vi "SSL Geometry Data.vi"(5 "Version":string(combo)="Auto", 7 "Optional":bool, 8 "error in":errorcluster, 9 "Array":u8[](array[numeric]) format="%02x") -> (0 "error out":errorcluster, 2 "Geometry Camera Calibration":T1, 3 "Field Size":T2)   [LabVIEW 2017]
uses:
  SSL Geometry Camera Calibration.ctl
  Varint Decoder uint32.vi
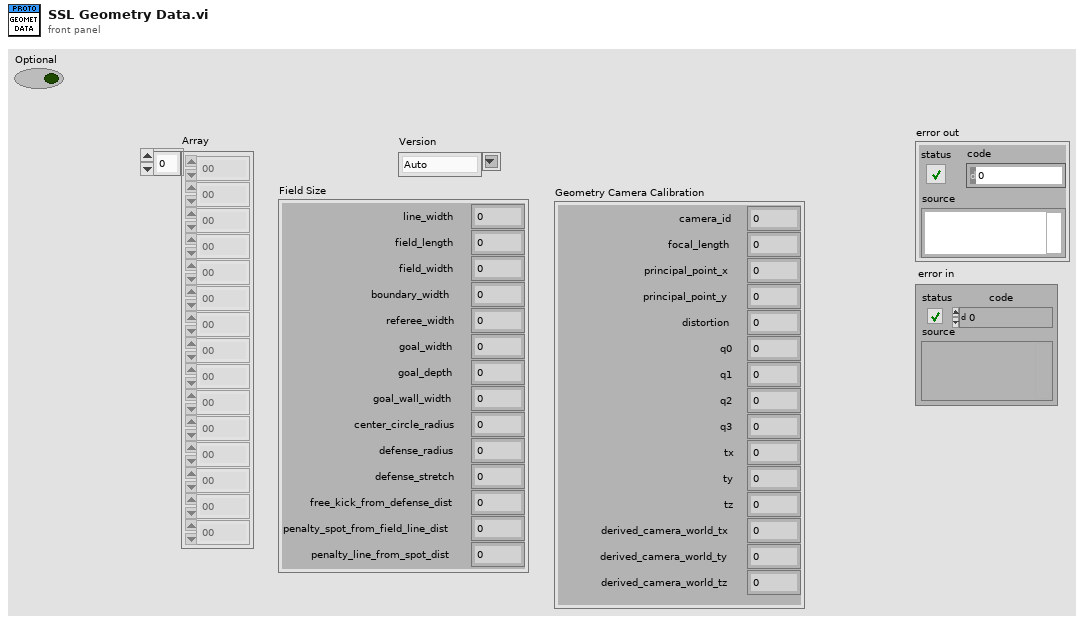
[diagram p1: front panel]
types:
  T1 = typedef "SSL Geometry Camera Calibration.ctl" = cluster{"camera_id":u32, "focal_length":sgl, "principal_point_x":sgl, "principal_point_y":sgl, "distortion":sgl, "q0":sgl, "q1":sgl, "q2":sgl, "q3":sgl, "tx":sgl, "ty":sgl, "tz":sgl, "derived_camera_world_tx":sgl, "derived_camera_world_ty":sgl, "derived_camera_world_tz":sgl}
  T2 = cluster{"line_width":u32, "field_length":u32, "field_width":u32, "boundary_width":u32, "referee_width":u32, "goal_width":u32, "goal_depth":u32, "goal_wall_width":u32, "center_circle_radius":u32, "defense_radius":u32, "defense_stretch":u32, "free_kick_from_defense_dist":u32, "penalty_spot_from_field_line_dist":u32, "penalty_line_from_spot_dist":u32}
  T3 = cluster{"[0]":sgl, "[1]":sgl, "[2]":sgl, "[3]":sgl, "[4]":sgl, "[5]":sgl, "[6]":sgl, "[7]":sgl, "[8]":sgl, "[9]":sgl, "[10]":sgl, "[11]":sgl, "[12]":sgl, "[13]":sgl, "[14]":sgl}
  T4 = cluster{"[0]":u32, "[1]":u32, "[2]":u32, "[3]":u32, "[4]":u32, "[5]":u32, "[6]":u32, "[7]":u32, "[8]":u32, "[9]":u32, "[10]":u32, "[11]":u32, "[12]":u32, "[13]":u32}
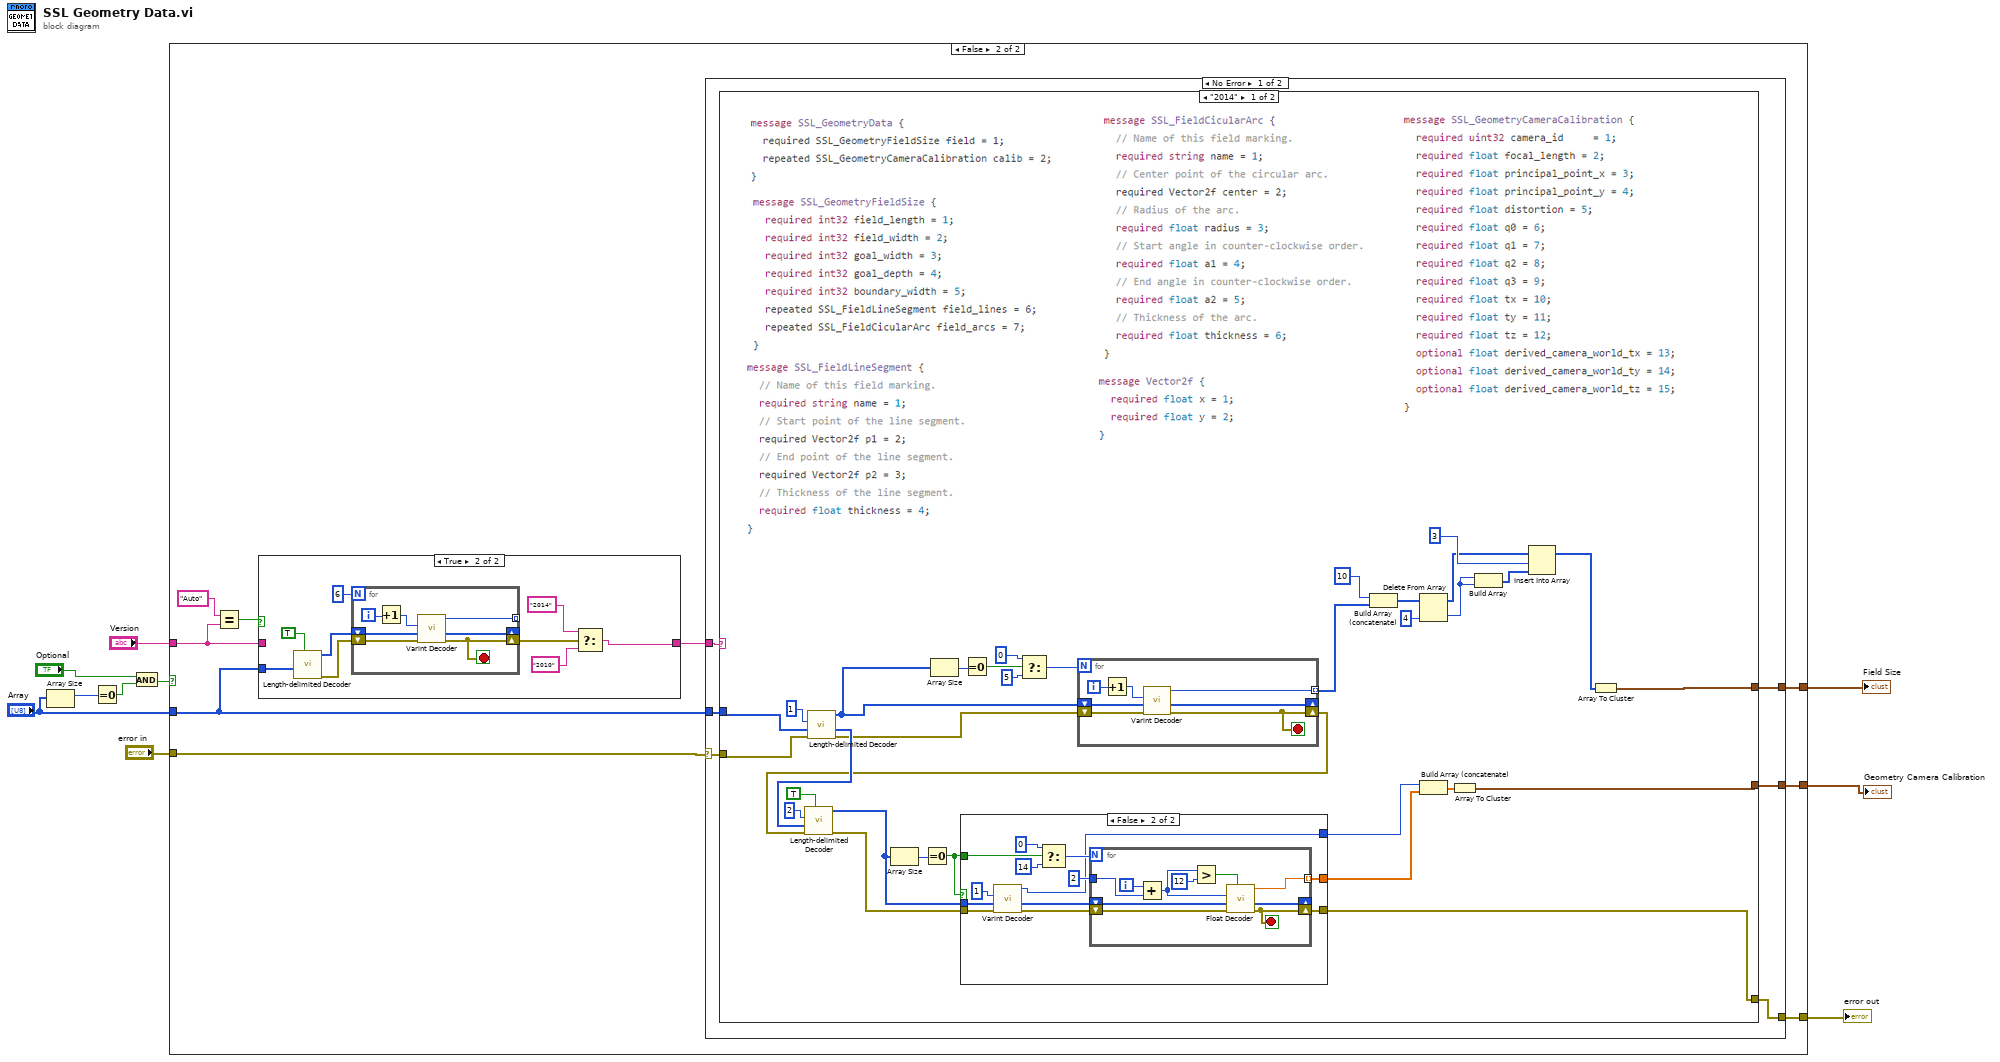
[diagram p0: block diagram]
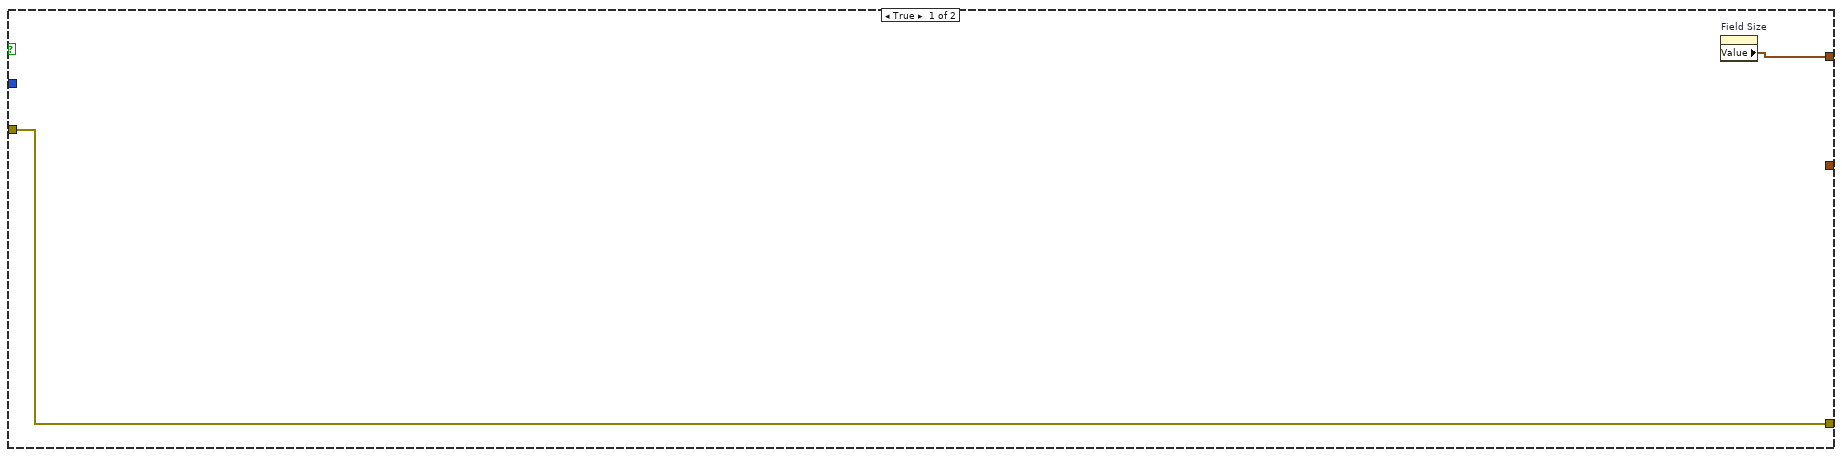
[diagram p2: hidden frame]
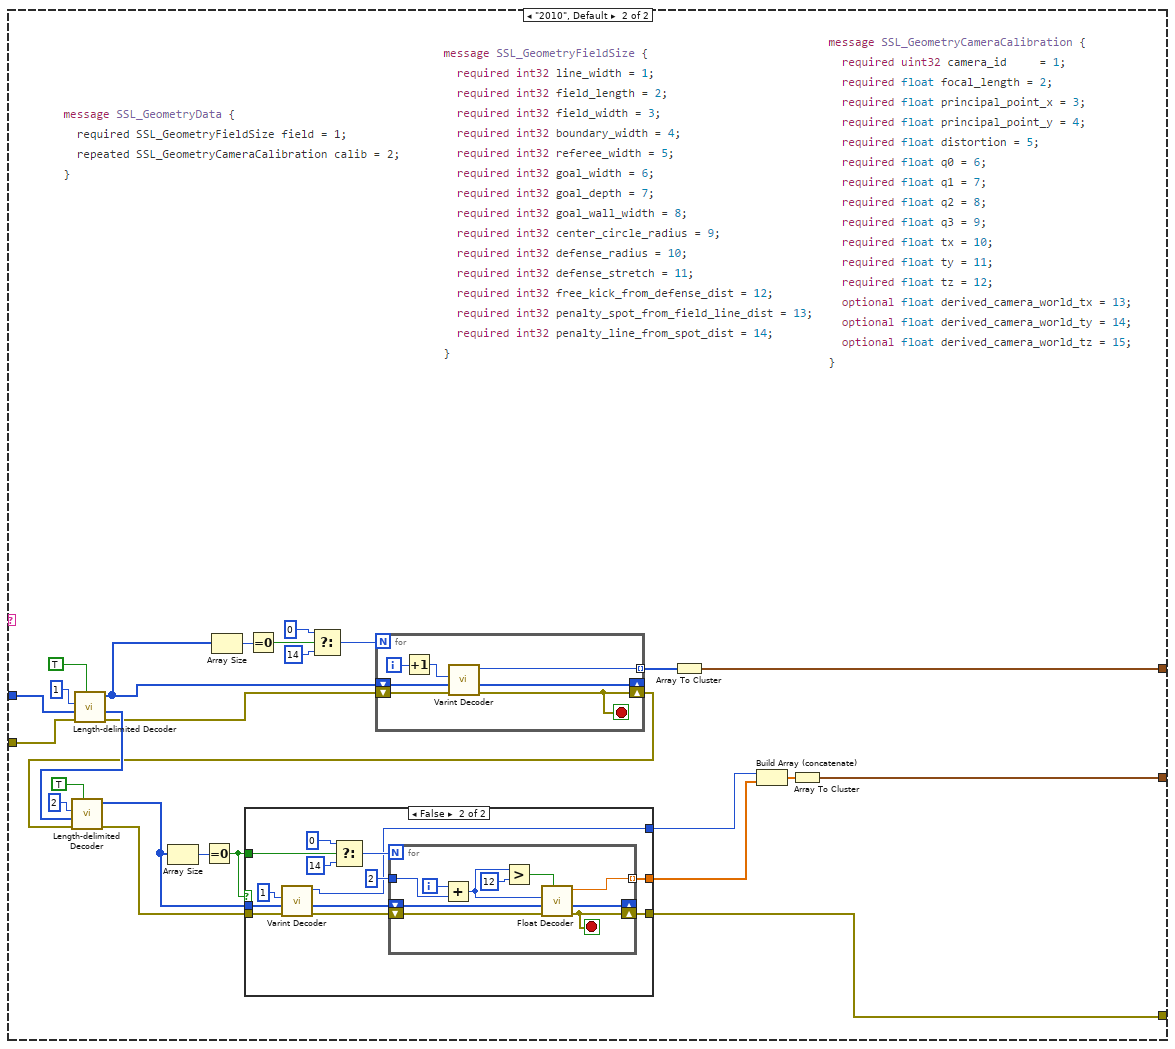
[diagram p5: hidden frame]
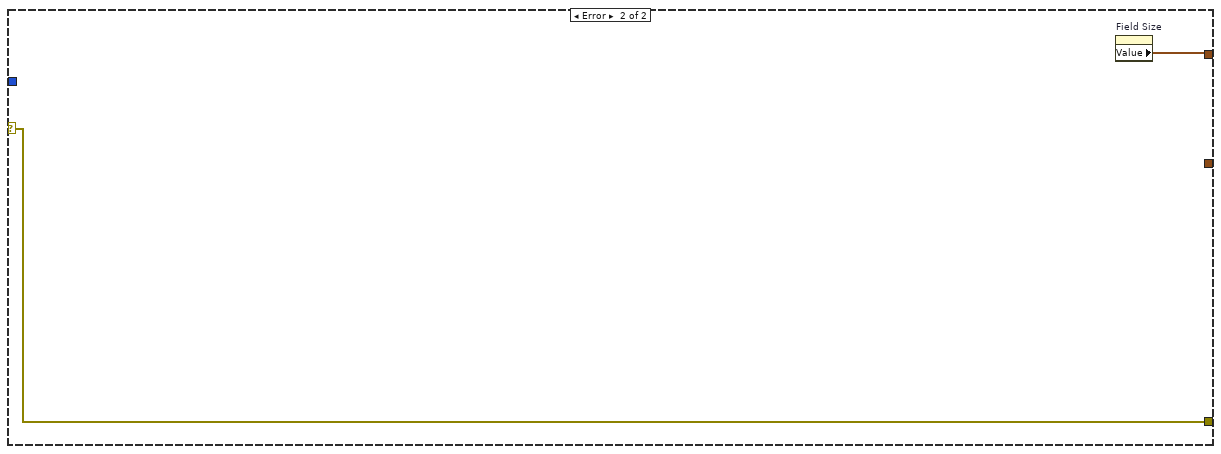
[diagram p7: hidden frame]
diagram:
  n1 = Array Size(array="Array") -> (size(s)=w4:i32)
  n2 = Equal To 0?(x=w4) -> (x = 0?=w5:bool)
  n3 = And(x="Optional", y=w5) -> (x .and. y?=w6:bool)
  n4 = case shown="False" w6 {
    tunnel: "error in" -> [w12 w21]
    tunnel: [w12 w20] -> w9
    tunnel: "Array" -> [_ w13]
    tunnel: "Version" -> [_ w15]
    tunnel: [w11 w19] -> w2
    tunnel: [_ w18] -> w1
    frame True {
      n5 = property on="Field Size" class="Clust (strict)"() -> ("Value"=w11:T2)  [unwired: 2 in, 2 out]
    }
    frame False {
      n6 = Equal?(x="Auto", y=w15) -> (x = y?=w16:bool)
      n7 = case shown="True" w16 {
        tunnel: w15 -> [w22 _]
        tunnel: [w22 w25] -> w14
        tunnel: w13 -> [_ w31]
        frame False {
        }
        frame True {
          n8 = call "Length-delimited Decoder.vi"("Optional"=TRUE, "Array"=w31) -> ("error out"=w29:errorcluster, "Length-delimited"=w30:u8[])  [unwired: 6 in, 2 out]
          n9 = for {
            N: 6 -> [_]
            tunnel: [w38] -> _ mode=indexing
            shift-right: [w37] -> _
            shift-left: w30 -> [w33]
            shift-right: [w35] -> w26
            shift-left: w29 -> [w36]
            i -> [w34]
            stop <- w35 stop-if-true
            n10 = Increment(x=w34) -> (x+1=w32:i32)
            n11 = call-poly "Varint Decoder.vi"("error in (no error)"=w36, "Array"=w33, "Key"=w32) -> ("error out"=w35:errorcluster, "array w/ subset deleted"=w37:u8[], "Varint"=w38:u32)  [unwired: 5 in, 1 out]
          }
          n12 = Select(t="2014" ("x"), s=w26, f="2010" ("x")) -> (s? t:f=w25:string)
        }
      }
      n13 = case shown="No Error" w21 {
        selector: w21 -> [w44 w167]
        tunnel: [w43 w167] -> w20
        tunnel: w13 -> [w42 _]
        tunnel: w14 -> [w41 _]
        tunnel: [w40 w166] -> w19
        tunnel: [w39 _] -> w18
        frame No Error {
          n14 = case shown="\"2014\"" w41 {
            tunnel: w44 -> [w57 w134]
            tunnel: [w56 w123] -> w43
            tunnel: w42 -> [w58 w116]
            tunnel: [w55 w110] -> w40
            tunnel: [w54 w109] -> w39
            frame "2014" {
              n15 = call "Length-delimited Decoder.vi"("error in (no error)"=w57, "Array"=w58, "Key"=1) -> ("error out"=w66:errorcluster, "array w/ subset deleted"=w68:u8[], "Length-delimited"=w75:u8[])  [unwired: 5 in, 1 out]
              n16 = Array Size(array=w75) -> (size(s)=w74:i32)
              n17 = Equal To 0?(x=w74) -> (x = 0?=w73:bool)
              n18 = Select(t=0, s=w73, f=5) -> (s? t:f=w70:i32)
              n19 = for {
                N: w70 -> [_]
                tunnel: [w108] -> w52 mode=indexing
                shift-right: [w107] -> _
                shift-left: w75 -> [w103]
                shift-right: [w105] -> w65
                shift-left: w66 -> [w106]
                i -> [w104]
                stop <- w105 stop-if-true
                n20 = Increment(x=w104) -> (x+1=w102:i32)
                n21 = call-poly "Varint Decoder.vi"("error in (no error)"=w106, "Array"=w103, "Key"=w102) -> ("error out"=w105:errorcluster, "array w/ subset deleted"=w107:u8[], "Varint"=w108:u32)  [unwired: 5 in, 1 out]
              }
              n22 = call "Length-delimited Decoder.vi"("Optional"=TRUE, "error in (no error)"=w65, "Array"=w68, "Key"=2) -> ("error out"=w64:errorcluster, "Length-delimited"=w59:u8[])  [unwired: 4 in, 2 out]
              n23 = Array Size(array=w59) -> (size(s)=w69:i32)
              n24 = Equal To 0?(x=w69) -> (x = 0?=w63:bool)
              n25 = case shown="False" w63 {
                tunnel: w63 -> [_ w91]
                tunnel: [w78 w87] -> w56
                tunnel: [_ w84] -> w61
                tunnel: w64 -> [w78 w82]
                tunnel: w59 -> [_ w81]
                tunnel: [_ w79] -> w62
                frame True {
                }
                frame False {
                  n26 = call-poly "Varint Decoder.vi"("error in (no error)"=w82, "Array"=w81, "Key"=1) -> ("error out"=w83:errorcluster, "array w/ subset deleted"=w86:u8[], "Varint"=w79:u32)  [unwired: 5 in, 1 out]
                  n27 = Select(t=0, s=w91, f=14) -> (s? t:f=w88:i32)
                  n28 = for {
                    N: w88 -> [_]
                    tunnel: [w94] -> w84 mode=indexing
                    shift-right: [w101] -> _
                    shift-left: w86 -> [w93]
                    shift-right: [w99] -> w87
                    shift-left: w83 -> [w100]
                    tunnel: 2 ("y") -> [w95]
                    i -> [w97]
                    stop <- w99 stop-if-true
                    n29 = Add(x=w97, y=w95) -> (x+y=w96:i32)
                    n30 = Greater?(x=w96, y=12) -> (0:w92:bool)
                    n31 = call "Float Decoder.vi"("Optional"=w92, "error in (no error)"=w100, "Array"=w93, "Key"=w96) -> ("error out"=w99:errorcluster, "array w/ subset deleted"=w101:u8[], "Float"=w94:sgl)  [unwired: 4 in, 1 out]
                  }
                }
              }
              n32 = Build Array (concatenate)(u32 10 ("element"), w52) -> (w51:u32[])
              n33 = Delete From Array(array=w51, index=4) -> (deleted portion=w49:u32, array with subset deleted=w47:u32[])  [unwired: 1 in]
              n34 = Build Array (concatenate)(w62, w61) -> (w60:sgl[])
              n35 = Array To Cluster(array=w60) -> (cluster=w54:T3)
              n36 = Build Array(w49, w49) -> (w48:u32[])
              n37 = Insert Into Array(array=w47, index=3, new element=w48) -> (w45:u32[])
              n38 = Array To Cluster(array=w45) -> (cluster=w55:T4)
            }
            frame "2010", Default {
              n39 = call "Length-delimited Decoder.vi"("Optional"=TRUE, "error in (no error)"=w134, "Array"=w116, "Key"=1) -> ("error out"=w120:errorcluster, "array w/ subset deleted"=w122:u8[], "Length-delimited"=w131:u8[])  [unwired: 4 in, 1 out]
              n40 = Array Size(array=w131) -> (size(s)=w130:i32)
              n41 = Equal To 0?(x=w130) -> (x = 0?=w129:bool)
              n42 = Select(t=0, s=w129, f=14) -> (s? t:f=w126:i32)
              n43 = for {
                N: w126 -> [_]
                tunnel: [w165] -> w125 mode=indexing
                shift-right: [w164] -> _
                shift-left: w131 -> [w160]
                shift-right: [w162] -> w119
                shift-left: w120 -> [w163]
                i -> [w161]
                stop <- w162 stop-if-true
                n44 = Increment(x=w161) -> (x+1=w159:i32)
                n45 = call-poly "Varint Decoder.vi"("error in (no error)"=w163, "Array"=w160, "Key"=w159) -> ("error out"=w162:errorcluster, "array w/ subset deleted"=w164:u8[], "Varint"=w165:u32)  [unwired: 5 in, 1 out]
              }
              n46 = call "Length-delimited Decoder.vi"("Optional"=TRUE, "error in (no error)"=w119, "Array"=w122, "Key"=2) -> ("error out"=w117:errorcluster, "Length-delimited"=w111:u8[])  [unwired: 4 in, 2 out]
              n47 = Array Size(array=w111) -> (size(s)=w124:i32)
              n48 = Equal To 0?(x=w124) -> (x = 0?=w115:bool)
              n49 = case shown="False" w115 {
                tunnel: w115 -> [_ w148]
                tunnel: [w135 w144] -> w123
                tunnel: [_ w141] -> w113
                tunnel: w117 -> [w135 w139]
                tunnel: w111 -> [_ w138]
                tunnel: [_ w136] -> w114
                frame True {
                }
                frame False {
                  n50 = call-poly "Varint Decoder.vi"("error in (no error)"=w139, "Array"=w138, "Key"=1) -> ("error out"=w140:errorcluster, "array w/ subset deleted"=w143:u8[], "Varint"=w136:u32)  [unwired: 5 in, 1 out]
                  n51 = Select(t=0, s=w148, f=14) -> (s? t:f=w145:i32)
                  n52 = for {
                    N: w145 -> [_]
                    tunnel: [w151] -> w141 mode=indexing
                    shift-right: [w158] -> _
                    shift-left: w143 -> [w150]
                    shift-right: [w156] -> w144
                    shift-left: w140 -> [w157]
                    tunnel: 2 ("y") -> [w152]
                    i -> [w154]
                    stop <- w156 stop-if-true
                    n53 = Add(x=w154, y=w152) -> (x+y=w153:i32)
                    n54 = Greater?(x=w153, y=12) -> (0:w149:bool)
                    n55 = call "Float Decoder.vi"("Optional"=w149, "error in (no error)"=w157, "Array"=w150, "Key"=w153) -> ("error out"=w156:errorcluster, "array w/ subset deleted"=w158:u8[], "Float"=w151:sgl)  [unwired: 4 in, 1 out]
                  }
                }
              }
              n56 = Array To Cluster(array=w125) -> (cluster=w110:T4)
              n57 = Build Array (concatenate)(w114, w113) -> (w112:sgl[])
              n58 = Array To Cluster(array=w112) -> (cluster=w109:T3)
            }
          }
        }
        frame Error {
          n59 = property on="Field Size" class="Clust (strict)"() -> ("Value"=w166:T2)  [unwired: 2 in, 2 out]
        }
      }
    }
  }
  "error out" <- w9
  "Field Size" <- w2
  "Geometry Camera Calibration" <- w1
